vi "(x,y) to XY (multiple).vi"(2 "[[(x,y)]]":cluster{"x":dbl, "y":dbl}[][](array[cluster]), 8 "error in (no error)":errorcluster) -> (0 "error out":errorcluster, 3 "XY-data out":cluster{"X-array":dbl[], "Y-array":dbl[]}[](array[cluster]) {"Y-array" format="%.2p"; "X-array" format="%.2p"})   [LabVIEW 2019, in "xy_utilities.lvlib"]
doc: "Convert <b>XY-data</b> (cluster of arrays of X and Y) to <b>(x,y)</b> coordinates (array of clusters of (x,y) values).\n\nWire data to the data input to determine the polymorphic instance to use or manually select the instance."
uses:
  xy_utilities.lvlib
  Initialize.vi
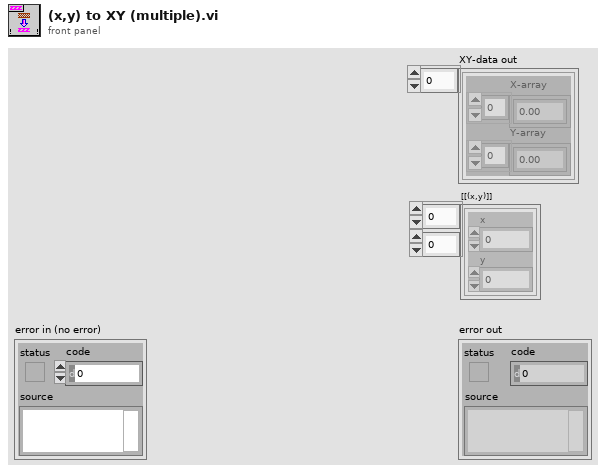
[diagram p1: front panel]
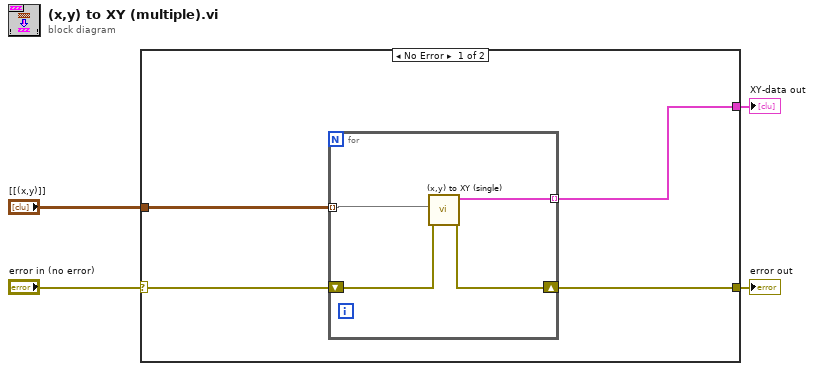
[diagram p0: block diagram]
diagram:
  n1 = case shown="No Error" "error in (no error)" {
    selector: "error in (no error)" -> [w8 w13]
    tunnel: [w7 w13] -> w3
    tunnel: [w5 _] -> w2
    tunnel: "[[(x,y)]]" -> [w6 _]
    frame No Error {
      n2 = for {
        shift-right: [w9] -> w7
        shift-left: w8 -> [w10]
        tunnel: w6 -> [w12] mode=indexing
        tunnel: [w11] -> w5 mode=indexing
        n3 = call "(x,y) to XY (single).vi"("error in (no error)"=w10, "[(x,y)]"=w12) -> ("error out"=w9:errorcluster, "XY-data out"=w11:cluster{"X-array":dbl[], "Y-array":dbl[]})  [unwired: 8 in]
      }
    }
    frame Error {
    }
  }
  "error out" <- w3
  "XY-data out" <- w2
